vi "Autonomous Independent.vi"() -> ()   [LabVIEW 2015]
doc: "This VI is called when autonomous begins, and will automatically be terminated when autonomous ends. You can carry out timed or sensor driven robot movement independently without needing to return to the caller."
uses:
  Robot Global Data.vi
  <vilib>/addons/control/pid/NI_PID_pid.lvlib
  <vilib>/addons/control/pid/pid.llb/PID (DBL).vi
  <vilib>/Rock Robotics/WPI/DriverStation/WPI_DriverStationRobotMode2.ctl
panel:
  out "time to goal":dbl
  # "Be sure to right-click and choose Data Operations>>Make Current Value default if you want to save the array values with the VI"
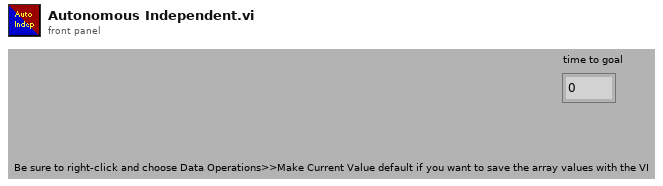
[diagram p1: front panel]
types:
  T1 = enum16{"Queen", "King", "Rook", "Knight", "Pawn"}
  T2 = typedef "WPI_DriverStationRobotMode2.ctl" = enum16{"Autonomous Disabled", "Autonomous Enabled", "Teleop Disabled", "Teleop Enabled", "Disconnected", "Finish", "Test Disabled", "Test Enabled"}
  T3 = typedef "TargetType.ctl" = enum16{"Not Hot", "Hot"}
  T4 = cluster{"Distance (ft)":dbl, "Target Center (-1 to 1)":cluster{"X":dbl, "Y":dbl}, "Left":bool, "State":T3, "Angle":dbl}
  T5 = typedef "WPI_MotorControlDeviceRef.ctl" = cluster{"DeviceStatus":errorcluster, "Type":enum16{"PWM", "CAN"}, "PWM":cluster{"Digital Module":T6, "PWM Channel":T7, "DeadBand":T8}, "CAN":cluster{"Device Number":u8, "Control Mode":T9, "Semaphore":T10, "Max Vout":dbl}, "Invert":bool, "TransformRef":T11, "InvTransformRef":T11}
  T6 = typedef "FPGA_TypedefDigitalModule.ctl" = enum16{"Digital Module 1", "Digital Module 2"}
  T7 = typedef "FPGA_DIOPWMChannel.ctl" = enum8{"PWM 1", "PWM 2", "PWM 3", "PWM 4", "PWM 5", "PWM 6", "PWM 7", "PWM 8", "PWM 9", "PWM 10", "Invalid"}
  T8 = typedef "WPI_PWMDeadband.ctl" = cluster{"Name":string, "maxPositivePwm":i32, "minPositivePwm":i32, "centerPwm":i32, "maxNegativePwm":i32, "minNegativePwm":i32, "angularRange":u16}
  T9 = typedef "WPI_CANJaguar_ControlMode.ctl" = enum8{"Percent VBus", "Current", "Speed", "Position", "Voltage"}
  T10 = typedef "Semaphore RefNum" = refnum<k1>
  T11 = typedef "WPI_PWMTransform_ConPane.ctl" = refnum<vi>
  T12 = cluster{"proportional gain (Kc)":dbl, "integral time (Ti, min)":dbl, "derivative time (Td, min)":dbl}
  T13 = typedef "WPI_GyroDevRef.ctl" = cluster{"DevStatus":errorcluster, "Analog Module":T14, "Analog Channel":T15, "Offset":dbl, "Gain (VoltsPerDegree/Second)":dbl}
  T14 = typedef "FPGA_TypedefAnalogModule.ctl" = enum16{"Analog Module 1", "Analog Module 2"}
  T15 = typedef "FPGA_AIChannel.ctl" = enum8{"AI 1", "AI 2", "AI 3", "AI 4", "AI 5", "AI 6", "AI 7", "AI 8", "Invalid"}
  T16 = typedef "WPI_EncoderDevRef.ctl" = cluster{"DevStatus":errorcluster, "EncoderIndex":T17, "CounterIndex":T18, "DistancePerCount":dbl, "Decoding Type":T19}
  T17 = typedef "FPGA_EncoderIdx.ctl" = enum8{"Enc 0", "Enc 1", "Enc 2", "Enc 3", "Invalid"}
  T18 = typedef "FPGA_CounterCtrSystemIndex.ctl" = enum8{"Ctr 0", "Ctr 1", "Ctr 2", "Ctr 3", "Ctr 4", "Ctr 5", "Ctr 6", "Ctr 7", "Invalid"}
  T19 = typedef "WPI_EncoderType.ctl" = enum16{"1x", "2x", "4x"}
  T20 = cluster{"Distance 1":dbl, "Angle":dbl, "Distance 2":dbl}
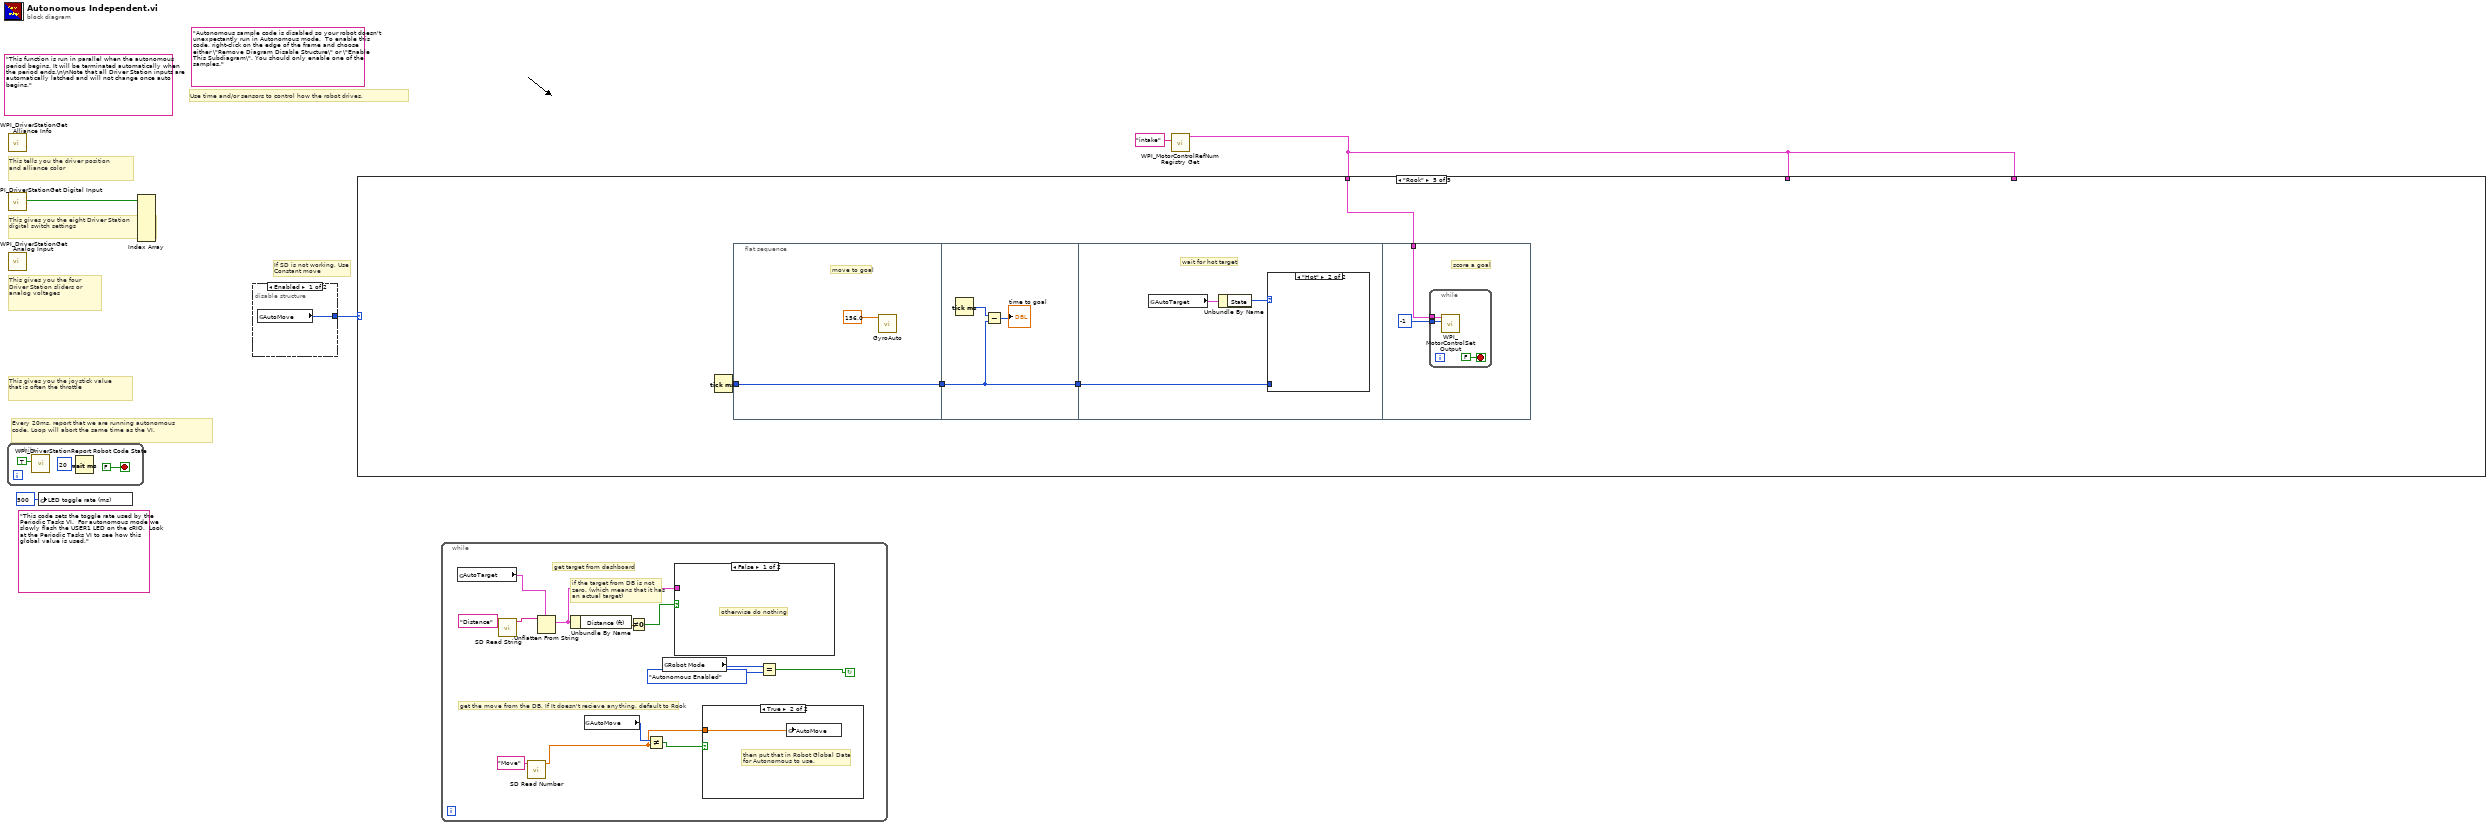
[diagram p0: block diagram]
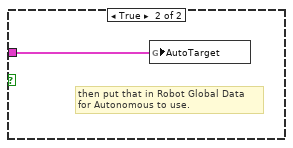
[diagram p3: hidden frame]
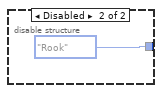
[diagram p4: hidden frame]
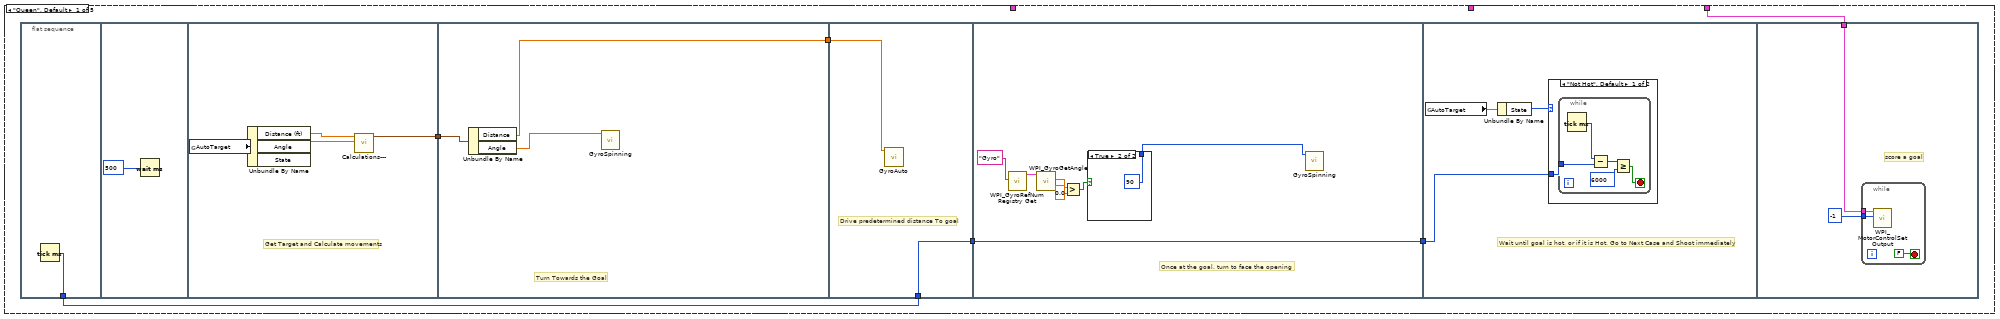
[diagram p5: hidden frame]
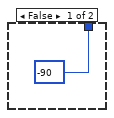
[diagram p6: hidden frame]
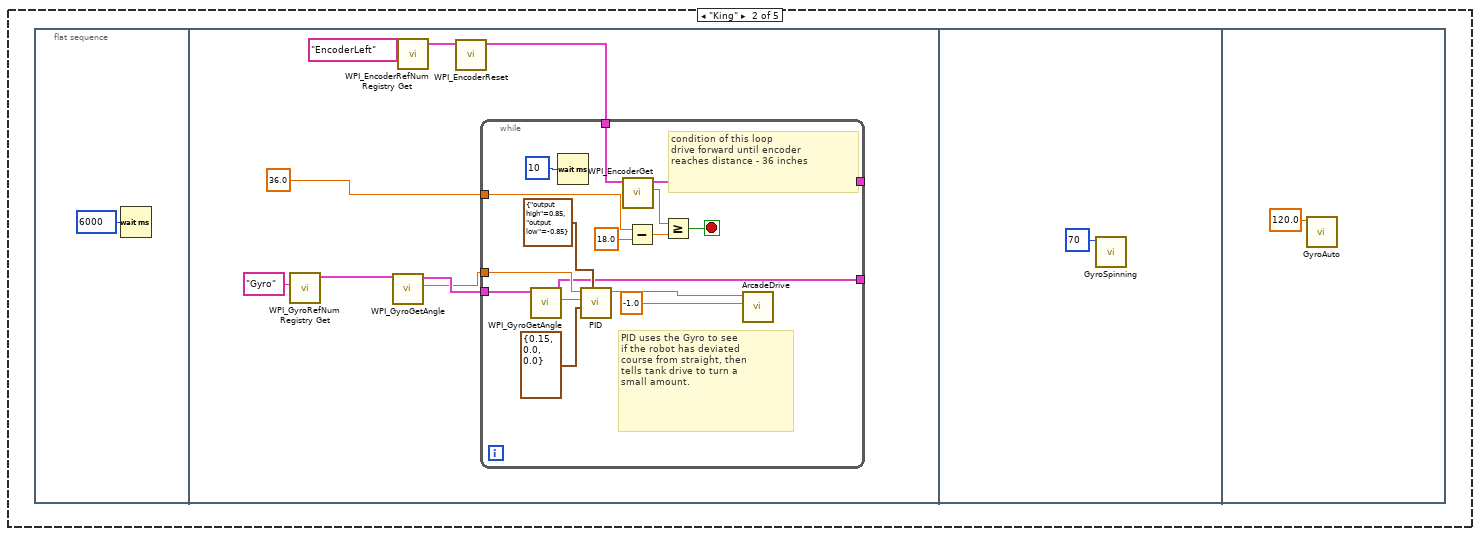
[diagram p8: hidden frame]
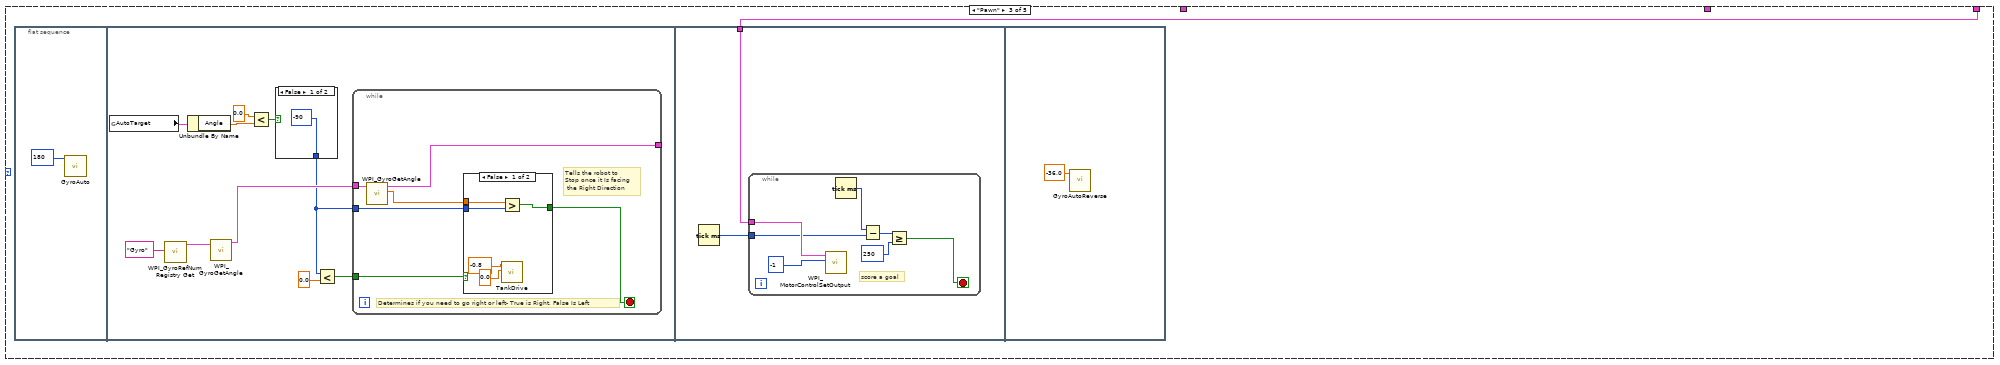
[diagram p9: hidden frame]
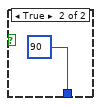
[diagram p10: hidden frame]
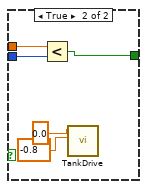
[diagram p11: hidden frame]
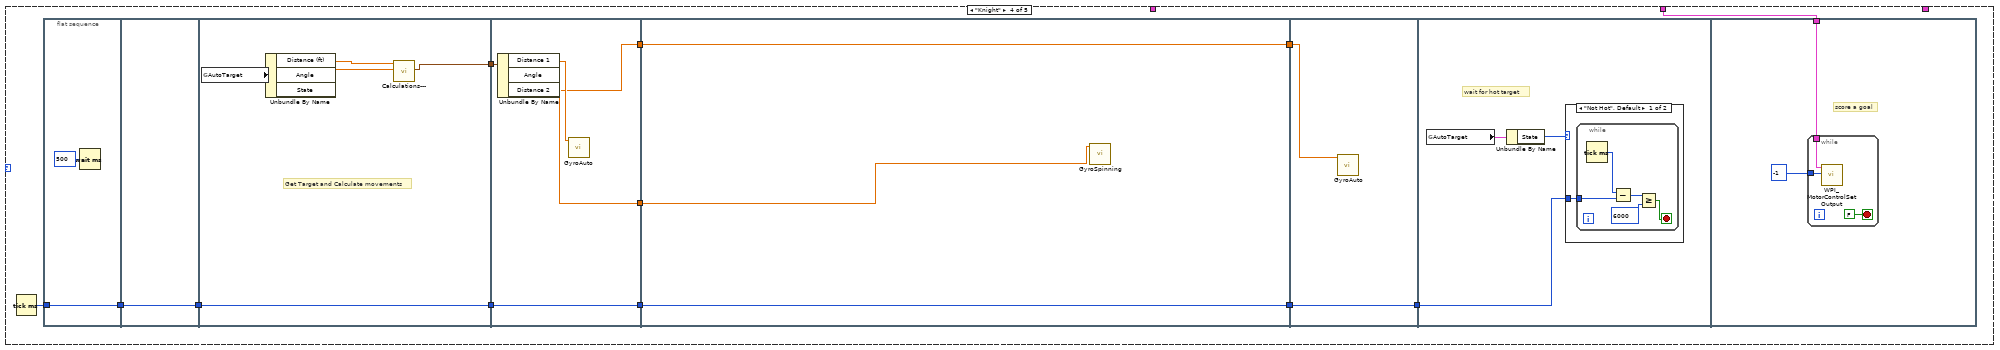
[diagram p12: hidden frame]
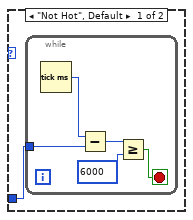
[diagram p14: hidden frame]
diagram:
  (unwired) "This code sets the toggle rate used by the Periodic Tasks VI.  For autonomous mode we slowly flash the USER1 LED on the cRIO.  Look at the Periodic Tasks VI to see how this global value is used."
  (unwired) "Autonomous sample code is disabled so your robot doesn't unexpectantly run in Autonomous mode.  To enable this code, right-click on the edge of the frame and choose either \"Remove Diagram Disable Structure\" or \"Enable This Subdiagram\". You should only enable one of the samples."
  (unwired) "This function is run in parallel when the autonomous period begins. It will be terminated automatically when the period ends.\n\nNote that all Driver Station inputs are automatically latched and will not change once auto begins."
  # "If SD is not working, Use \nConstant move"
  # "Every 20ms, report that we are running autonomous\ncode. Loop will abort the same time as the VI."
  # "This gives you the joystick value\nthat is often the throttle"
  # "Use time and/or sensors to control how the robot drives."
  # "This tells you the driver position\nand alliance color"
  # "This gives you the eight Driver Station\ndigital switch settings"
  # "This gives you the four\nDriver Station sliders or\nanalog voltages"
  n1 = while {
    stop <- FALSE stop-if-true
    n2 = call <vilib>:"WPI_DriverStationReport Robot Code State.vi"("Autonomous"=TRUE) -> ()  [unwired: 10 in, 1 out]
    n3 = Wait (ms)(milliseconds to wait=u32 20) -> ()  [unwired: 1 out]
  }
  n4 = call <vilib>:"WPI_DriverStationGet Alliance Info.vi"() -> ()  [unwired: 12 out]
  n5 = call <vilib>:"WPI_DriverStationGet Digital Input.vi"() -> ("Driver Station Digital Input (1-8)"=w5:bool[])  [unwired: 11 out]
  n6 = call <vilib>:"WPI_DriverStationGet Analog Input.vi"() -> ()  [unwired: 12 out]
  n7 = global write "Robot Global Data.vi" "LED toggle rate (ms)"(u32 500 ("LED ms toggle rate")) -> ()
  n8 = Index Array(array=w5) -> ()  [unwired: 8 in, 8 out]
  n9 = disable-structure shown="Enabled" {
    disable-tunnel: [w9 T1."Rook" ("AutoMove")] -> w1
    frame Enabled {
      n10 = global read "Robot Global Data.vi" "AutoMove"() -> (w9:T1)
    }
    frame Disabled {
    }
  }
  n11 = while {
    stop <- w15 continue-if-true
    # "get the move from the DB. If It doesn't recieve anything, default to Rook"
    # "if the target from DB is not\nzero. (which means that it has\nan actual target)"
    # "get target from dashboard"
    n12 = global read "Robot Global Data.vi" "AutoTarget"() -> (w21:T4)
    n13 = call <vilib>:"SD Read String.vi"("Name"="Distance") -> ("String"=w22:string)  [unwired: 8 in, 2 out]
    n14 = call <vilib>:"SD Read Number.vi"("Name"="Move") -> ("Numeric"=w11:dbl)  [unwired: 8 in, 2 out]
    n15 = Unflatten From String(type=w21, binary string=w22) -> (value=w19:T4)  [unwired: 3 in, 2 out]
    n16 = Unbundle By Name(w19) -> ("Distance (ft)"=w18:dbl)
    n17 = global read "Robot Global Data.vi" "AutoMove"() -> (w12:T1)
    n18 = Not Equal To 0?(x=w18) -> (x != 0?=w20:bool)
    n19 = Not Equal?(x=w12, y=w11) -> (x != y?=w13:bool)
    n20 = global read "Robot Global Data.vi" "Robot Mode"() -> (w17:T2)
    n21 = case shown="False" w20 {
      tunnel: w19 -> [_ w25]
      frame False {
        # "otherwise do nothing"
      }
      frame True {
        # "then put that in Robot Global Data \nfor Autonomous to use."
        n22 = global write "Robot Global Data.vi" "AutoTarget"(w25) -> ()
      }
    }
    n23 = case shown="True" w13 {
      tunnel: w11 -> [_ w24]
      frame False {
        # "otherwise do nothing"
      }
      frame True {
        # "then put that in Robot Global Data \nfor Autonomous to use."
        n24 = global write "Robot Global Data.vi" "AutoMove"(w24) -> ()
      }
    }
    n25 = Equal?(x=w17, y=WPI_DriverStationRobotMode2."Autonomous Enabled") -> (x = y?=w15:bool)
  }
  n26 = call <vilib>:"WPI_MotorControlRefNum Registry Get.vi"("refnum name"="intake") -> ("MotorControlDevRef"=w2:T5)  [unwired: 9 in, 1 out]
  n27 = case shown="\"Rook\"" w1 {
    tunnel: w2 -> [_ _ _ _ w179]
    tunnel: w2 -> [w27 _ w93 _ _]
    tunnel: w2 -> [_ _ _ w135 _]
    frame "Queen", Default {
      n28 = flat-sequence {
        tunnel: [w32] -> w26
        tunnel: [w34] -> w31
        tunnel: w31 -> [w40]
        tunnel: [w39] -> w30
        tunnel: w30 -> [w42]
        tunnel: [w41] -> w29
        tunnel: w26 -> [w41]
        tunnel: w29 -> [w49]
        tunnel: [w49] -> w28
        tunnel: w28 -> [w52]
        tunnel: w27 -> [w61]
        frame #0 {
          n29 = Tick Count (ms)() -> (millisecond timer value=w32:u32)
        }
        frame #1 {
          n30 = Wait (ms)(milliseconds to wait=u32 500) -> ()  [unwired: 1 out]
        }
        frame #2 {
          # "Get Target and Calculate movements"
          n31 = global read "Robot Global Data.vi" "AutoTarget"() -> (w37:T4)
          n32 = Unbundle By Name(w37) -> ("Distance (ft)"=w36:dbl, "Angle"=w35:dbl)  [unwired: 1 out]
          n33 = call "Calculations---.vi"("angle"=w35, "distance"=w36) -> ("Queen"=w34:cluster{"Distance":dbl, "Angle":dbl})  [unwired: 8 in, 1 out]
        }
        frame #3 {
          # "Turn Towards the Goal"
          n34 = Unbundle By Name(w40) -> ("Distance"=w39:dbl, "Angle"=w38:dbl)
          n35 = call "GyroSpinning.vi"("Angle"=w38) -> ()  [unwired: 11 in]
        }
        frame #4 {
          # "Drive predetermined distance To goal"
          n36 = call "GyroAuto.vi"("Distance(In)"=w42) -> ()  [unwired: 11 in]
        }
        frame #5 {
          # "Once at the goal, turn to face the opening"
          n37 = call <vilib>:"WPI_GyroRefNum Registry Get.vi"("refnum name"="Gyro") -> ("GyroDevRef"=w44:T13)  [unwired: 9 in, 1 out]
          n38 = call <vilib>:"WPI_GyroGetAngle.vi"("GyroDevRef"=w44) -> ("Angle"=w48:dbl)  [unwired: 7 in, 3 out]
          n39 = Greater?(x=w48, y=0.0) -> (0:w46:bool)
          n40 = case shown="True" w46 {
            tunnel: [-90 90] -> w45
            frame False {
            }
            frame True {
            }
          }
          n41 = call "GyroSpinning.vi"("Angle"=w45) -> ()  [unwired: 11 in]
        }
        frame #6 {
          # "Wait until goal is hot, or if it is Hot, Go to Next Case and Shoot immediately"
          n42 = global read "Robot Global Data.vi" "AutoTarget"() -> (w54:T4)
          n43 = Unbundle By Name(w54) -> ("State"=w53:T3)
          n44 = case shown="\"Not Hot\", Default" w53 {
            tunnel: w52 -> [w55 _]
            frame "Not Hot", Default {
              n45 = while {
                tunnel: w55 -> [w56]
                stop <- w57 stop-if-true
                n46 = Tick Count (ms)() -> (millisecond timer value=w60:u32)
                n47 = Subtract(x=w60, y=w56) -> (x-y=w59:u32)
                n48 = Greater Or Equal?(x=w59, y=6000) -> (x >= y?=w57:bool)
              }
            }
            frame "Hot" {
            }
          }
        }
        frame #7 {
          # "score a goal"
          n49 = while {
            tunnel: -1 -> [w65]
            tunnel: w61 -> [w64]
            stop <- FALSE stop-if-true
            n50 = call <vilib>:"WPI_MotorControlSetOutput.vi"("Output"=w65, "MotorControlDevRef"=w64) -> ()  [unwired: 7 in, 3 out]
          }
        }
      }
    }
    frame "King" {
      n51 = flat-sequence {
        frame #0 {
          n52 = Wait (ms)(milliseconds to wait=u32 6000) -> ()  [unwired: 1 out]
        }
        frame #1 {
          n53 = call <vilib>:"WPI_GyroRefNum Registry Get.vi"("refnum name"="Gyro") -> ("GyroDevRef"=w72:T13)  [unwired: 9 in, 1 out]
          n54 = call <vilib>:"WPI_GyroGetAngle.vi"("GyroDevRef"=w72) -> ("Angle"=w70:dbl, "GyroDevRef"=w71:T13)  [unwired: 7 in, 2 out]
          n55 = call <vilib>:"WPI_EncoderRefNum Registry Get.vi"("refnum name"="EncoderLeft") -> ("EncoderDevRef"=w69:T16)  [unwired: 9 in, 1 out]
          n56 = call <vilib>:"WPI_EncoderReset.vi"("EncoderDevRef"=w69) -> ("EncoderDevRef"=w68:T16)  [unwired: 9 in, 1 out]
          n57 = while {
            tunnel: 36.0 ("Distance(In)") -> [w81]
            tunnel: w68 -> [w84]
            tunnel: [w80] -> _
            tunnel: [w75] -> _
            tunnel: w70 -> [w79]
            tunnel: w71 -> [w78]
            stop <- w90 stop-if-true
            # "PID uses the Gyro to see \nif the robot has deviated \ncourse from straight, then\ntells tank drive to turn a \nsmall amount."
            # "condition of this loop\ndrive forward until encoder \nreaches distance - 36 inches"
            n58 = call <vilib>:"WPI_GyroGetAngle.vi"("GyroDevRef"=w78) -> ("Angle"=w87:dbl, "GyroDevRef"=w75:T13)  [unwired: 7 in, 2 out]
            n59 = Wait (ms)(milliseconds to wait=10) -> ()  [unwired: 1 out]
            n60 = call-poly <vilib>:"PID.vi"("output range"=cluster{"output high":dbl, "output low":dbl} {"output high"=0.85, "output low"=-0.85}, "PID gains"=T12 {"proportional gain (Kc)"=0.15, "integral time (Ti, min)"=0.0, "derivative time (Td, min)"=0.0}, "process variable"=w87, "setpoint"=w79) -> ("output"=w76:dbl)  [unwired: 6 in, 1 out]
            n61 = call <vilib>:"WPI_EncoderGet.vi"("EncoderDevRef"=w84) -> ("Distance"=w86:dbl, "EncoderDevRef"=w80:T16)  [unwired: 5 in, 4 out]
            n62 = Subtract(x=w81, y=18.0) -> (x-y=w83:dbl)
            n63 = Greater Or Equal?(x=w86, y=w83) -> (x >= y?=w90:bool)
            n64 = call "ArcadeDrive.vi"("y"=-1.0, "x"=w76) -> ()  [unwired: 10 in]
          }
        }
        frame #2 {
          n65 = call "GyroSpinning.vi"("Angle"=70) -> ()  [unwired: 11 in]
        }
        frame #3 {
          n66 = call "GyroAuto.vi"("Distance(In)"=120.0) -> ()  [unwired: 11 in]
        }
      }
    }
    frame "Pawn" {
      n67 = flat-sequence {
        tunnel: w93 -> [w124]
        frame #0 {
          n68 = call "GyroAuto.vi"("Distance(In)"=180) -> ()  [unwired: 11 in]
        }
        frame #1 {
          n69 = global read "Robot Global Data.vi" "AutoTarget"() -> (w99:T4)
          n70 = call <vilib>:"WPI_GyroRefNum Registry Get.vi"("refnum name"="Gyro") -> ("GyroDevRef"=w103:T13)  [unwired: 9 in, 1 out]
          n71 = Unbundle By Name(w99) -> ("Angle"=w97:dbl)
          n72 = call <vilib>:"WPI_GyroGetAngle.vi"("GyroDevRef"=w103) -> ("GyroDevRef"=w104:T13)  [unwired: 7 in, 3 out]
          n73 = Less?(x=0.0, y=w97) -> (x < y?=w98:bool)
          n74 = case shown="False" w98 {
            tunnel: [-90 90] -> w95
            frame False {
            }
            frame True {
            }
          }
          n75 = Less?(x=w95, y=0.0) -> (x < y?=w100:bool)
          n76 = while {
            tunnel: w104 -> [w112]
            tunnel: [w109] -> _
            tunnel: w95 -> [w108]
            tunnel: w100 -> [w107]
            stop <- w110 stop-if-true
            # "Tells the robot to \nStop once it Is facing\n the Right Direction"
            # "Determines if you need to go right or left- True is Right, False Is Left"
            n77 = call <vilib>:"WPI_GyroGetAngle.vi"("GyroDevRef"=w112) -> ("Angle"=w111:dbl, "GyroDevRef"=w109:T13)  [unwired: 7 in, 2 out]
            n78 = case shown="False" w107 {
              tunnel: w111 -> [w117 w122]
              tunnel: [w116 w121] -> w110
              tunnel: w108 -> [w113 w118]
              frame False {
                n79 = call "TankDrive.vi"("right"=0.0, "left"=-0.8) -> ()  [unwired: 10 in]
                n80 = Greater?(x=w117, y=w113) -> (0:w116:bool)
              }
              frame True {
                n81 = Less?(x=w122, y=w118) -> (x < y?=w121:bool)
                n82 = call "TankDrive.vi"("right"=-0.8, "left"=0.0) -> ()  [unwired: 10 in]
              }
            }
          }
        }
        frame #2 {
          n83 = Tick Count (ms)() -> (millisecond timer value=w123:u32)
          n84 = while {
            tunnel: w124 -> [w131]
            tunnel: w123 -> [w125]
            stop <- w127 stop-if-true
            # "score a goal"
            n85 = call <vilib>:"WPI_MotorControlSetOutput.vi"("Output"=-1, "MotorControlDevRef"=w131) -> ()  [unwired: 7 in, 3 out]
            n86 = Tick Count (ms)() -> (millisecond timer value=w128:u32)
            n87 = Subtract(x=w128, y=w125) -> (x-y=w129:u32)
            n88 = Greater Or Equal?(x=w129, y=250) -> (x >= y?=w127:bool)
          }
        }
        frame #3 {
          n89 = call "GyroAutoReverse.vi"("distance(in)"=-36.0 ("Distance(In)")) -> ()  [unwired: 11 in]
        }
      }
    }
    frame "Knight" {
      n90 = Tick Count (ms)() -> (millisecond timer value=w136:u32)
      n91 = flat-sequence {
        tunnel: w136 -> [w146]
        tunnel: [w146] -> w134
        tunnel: w134 -> [w147]
        tunnel: [w147] -> w133
        tunnel: [w149] -> w144
        tunnel: [w148] -> w138
        tunnel: w133 -> [w148]
        tunnel: w144 -> [w157]
        tunnel: [w155] -> w143
        tunnel: [w154] -> w141
        tunnel: w138 -> [w153]
        tunnel: [w153] -> w137
        tunnel: w143 -> [w158]
        tunnel: [w160] -> w142
        tunnel: w141 -> [w160]
        tunnel: [w159] -> w139
        tunnel: w137 -> [w159]
        tunnel: w142 -> [w162]
        tunnel: [w161] -> w140
        tunnel: w139 -> [w161]
        tunnel: w140 -> [w163]
        tunnel: w135 -> [w172]
        frame #0 {
          n92 = Wait (ms)(milliseconds to wait=u32 500) -> ()  [unwired: 1 out]
        }
        frame #1 {
        }
        frame #2 {
          # "Get Target and Calculate movements"
          n93 = global read "Robot Global Data.vi" "AutoTarget"() -> (w152:T4)
          n94 = Unbundle By Name(w152) -> ("Distance (ft)"=w151:dbl, "Angle"=w150:dbl)  [unwired: 1 out]
          n95 = call "Calculations---.vi"("angle"=w150, "distance"=w151) -> ("Knight"=w149:T20)  [unwired: 8 in, 1 out]
        }
        frame #3 {
          n96 = Unbundle By Name(w157) -> ("Distance 1"=w156:dbl, "Angle"=w155:dbl, "Distance 2"=w154:dbl)
          n97 = call "GyroAuto.vi"("Distance(In)"=w156) -> ()  [unwired: 11 in]
        }
        frame #4 {
          n98 = call "GyroSpinning.vi"("Angle"=w158) -> ()  [unwired: 11 in]
        }
        frame #5 {
          n99 = call "GyroAuto.vi"("Distance(In)"=w162) -> ()  [unwired: 11 in]
        }
        frame #6 {
          # "wait for hot target"
          n100 = global read "Robot Global Data.vi" "AutoTarget"() -> (w165:T4)
          n101 = Unbundle By Name(w165) -> ("State"=w164:T3)
          n102 = case shown="\"Not Hot\", Default" w164 {
            tunnel: w163 -> [w166 _]
            frame "Not Hot", Default {
              n103 = while {
                tunnel: w166 -> [w167]
                stop <- w168 stop-if-true
                n104 = Tick Count (ms)() -> (millisecond timer value=w171:u32)
                n105 = Subtract(x=w171, y=w167) -> (x-y=w170:u32)
                n106 = Greater Or Equal?(x=w170, y=6000) -> (x >= y?=w168:bool)
              }
            }
            frame "Hot" {
            }
          }
        }
        frame #7 {
          # "score a goal"
          n107 = while {
            tunnel: -1 -> [w176]
            tunnel: w172 -> [w174]
            stop <- FALSE stop-if-true
            n108 = call <vilib>:"WPI_MotorControlSetOutput.vi"("Output"=w176, "MotorControlDevRef"=w174) -> ()  [unwired: 7 in, 3 out]
          }
        }
      }
    }
    frame "Rook" {
      n109 = Tick Count (ms)() -> (millisecond timer value=w180:u32)
      n110 = flat-sequence {
        tunnel: [w182] -> w178
        tunnel: w180 -> [w182]
        tunnel: w178 -> [w183]
        tunnel: [w183] -> w177
        tunnel: w177 -> [w186]
        tunnel: w179 -> [w195]
        frame #0 {
          # "move to goal"
          n111 = call "GyroAuto.vi"("Distance(In)"=156.0) -> ()  [unwired: 11 in]
        }
        frame #1 {
          n112 = Tick Count (ms)() -> (millisecond timer value=w184:u32)
          n113 = Subtract(x=w184, y=w183) -> (x-y=→"time to goal":u32)
        }
        frame #2 {
          # "wait for hot target"
          n114 = global read "Robot Global Data.vi" "AutoTarget"() -> (w188:T4)
          n115 = Unbundle By Name(w188) -> ("State"=w187:T3)
          n116 = case shown="\"Hot\"" w187 {
            tunnel: w186 -> [w189 _]
            frame "Not Hot", Default {
              n117 = while {
                tunnel: w189 -> [w194]
                stop <- w190 stop-if-true
                n118 = Tick Count (ms)() -> (millisecond timer value=w193:u32)
                n119 = Subtract(x=w193, y=w194) -> (x-y=w192:u32)
                n120 = Greater Or Equal?(x=w192, y=6000) -> (x >= y?=w190:bool)
              }
            }
            frame "Hot" {
            }
          }
        }
        frame #3 {
          # "score a goal"
          n121 = while {
            tunnel: -1 -> [w199]
            tunnel: w195 -> [w198]
            stop <- FALSE stop-if-true
            n122 = call <vilib>:"WPI_MotorControlSetOutput.vi"("Output"=w199, "MotorControlDevRef"=w198) -> ()  [unwired: 7 in, 3 out]
          }
        }
      }
    }
  }
